vi "DSF.Engine.Transceiver.Initialize.vi"(8 "error in (no error)":errorcluster, 9 "transceiver settings":T1, 10 "Transfer Groups Configurations":refnum<class "DSF.Shared.Configuration.Transfer Group.lvclass">[](array[class]), 11 "Transceiver in":refnum<class "DSF.Transceiver.GE Reflective Memory.lvclass">) -> (0 "error out":errorcluster, 3 "Transceiver out":refnum<class "DSF.Transceiver.GE Reflective Memory.lvclass">)   [LabVIEW 2017, in "DSF.Transceiver.GE Reflective Memory.lvlib" / "DSF.Transceiver.GE Reflective Memory.lvclass"]
uses:
  DSF.Transceiver.GE Reflective Memory.lvclass
  Built/Windows/Engine/DSF.Engine.lvlibp/Shared/Classes/Transfer Group/DSF.Shared.Configuration.Transfer Group.lvclass
  Built/Windows/Engine/DSF.Engine.lvlibp/DSF Configuration API/1.0.0/Public/Controls/DSF Settings Info.ctl
  Built/Windows/Engine/DSF.Engine.lvlibp/Engine/Classes/Transceiver/DSF.Engine.Transceiver.lvclass
  Built/Windows/Engine/DSF.Engine.lvlibp/DSF Configuration API/1.0.0/DSF Configuration API.lvlib
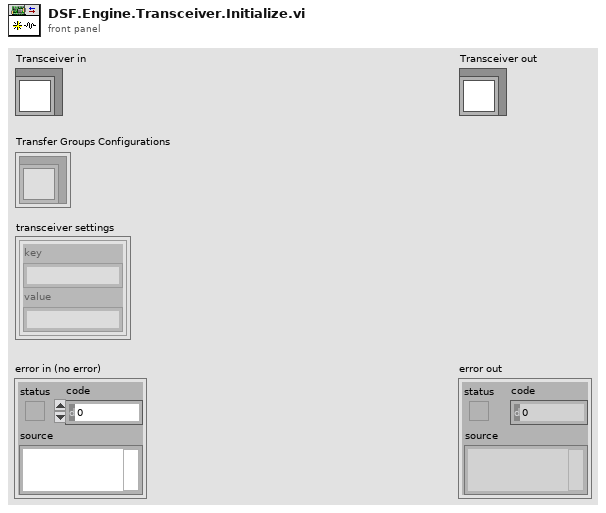
[diagram p1: front panel]
types:
  T1 = typedef "DSF.Engine.lvlibp/DSF Configuration API.lvlib/DSF Settings Info.ctl" = cluster{"key":string, "value":string}[]
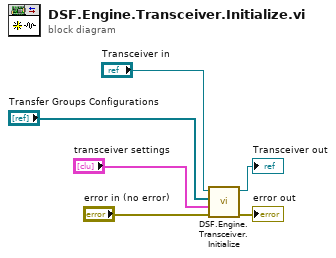
[diagram p0: block diagram]
diagram:
  n1 = call-parent "DSF.Engine.Transceiver.Initialize.vi"("error in (no error)"="error in (no error)", "transceiver settings"="transceiver settings", "Transfer Groups Configurations"="Transfer Groups Configurations", "Transceiver in"="Transceiver in") -> ("error out"=→"error out":errorcluster, "Transceiver out"=→"Transceiver out":refnum<class "DSF.Transceiver.GE Reflective Memory.lvclass">)  [unwired: 6 in]
